vi "Set Transfer Groups.vi"(6 "Async Tx Transfer Groups":refnum<class "Transfer Group.lvclass">[](array[class]), 8 "Async Rx Transfer Groups":refnum<class "Transfer Group.lvclass">[](array[class]), 9 "Inline Tx Transfer Groups":refnum<class "Transfer Group.lvclass">[](array[class]), 10 "Inline Rx Transfer Groups":refnum<class "Transfer Group.lvclass">[](array[class]), 11 "Mock Plugin in":refnum<class "Mock Plugin.lvclass">) -> (3 "Mock Plugin out":refnum<class "Mock Plugin.lvclass">)   [LabVIEW 2017, in "Mock Plugin.lvclass"]
uses:
  Mock Plugin.lvclass
  C:/github/data-sharing-framework/Data Sharing Framework Core/Engine/Classes/Plugin/Plugin.lvclass
  Engine/Classes/Transfer Group/Transfer Group.lvclass
  Engine/Classes/Plugin/Plugin.lvclass/Plugin.ctl
  Engine/Classes/Plugin/Plugin.lvclass
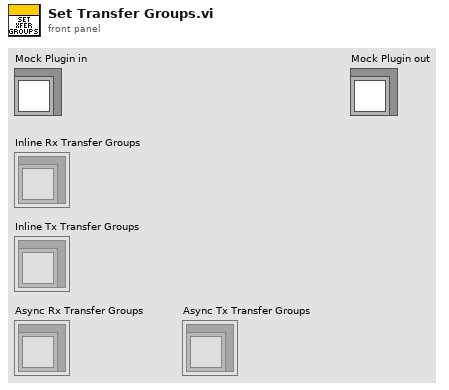
[diagram p1: front panel]
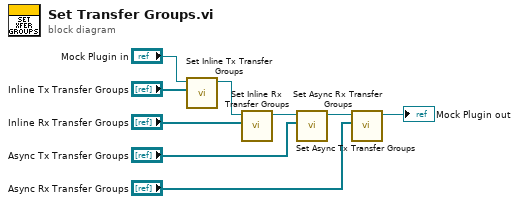
[diagram p0: block diagram]
diagram:
  n1 = call "Set Inline Tx Transfer Groups.vi"("Inline Tx Transfer Groups"="Inline Tx Transfer Groups", "Plugin in"="Mock Plugin in") -> ("Plugin out"=w7:refnum<class "Mock Plugin.lvclass">)  [unwired: 9 in]
  n2 = call "Set Inline Rx Transfer Groups.vi"("Inline Rx Transfer Groups"="Inline Rx Transfer Groups", "Plugin in"=w7) -> ("Plugin out"=w6:refnum<class "Mock Plugin.lvclass">)  [unwired: 9 in]
  n3 = call "Set Async Tx Transfer Groups.vi"("Async Tx Transfer Groups"="Async Tx Transfer Groups", "Plugin in"=w6) -> ("Plugin out"=w5:refnum<class "Mock Plugin.lvclass">)  [unwired: 9 in]
  n4 = call "Set Async Rx Transfer Groups.vi"("Async Rx Transfer Groups"="Async Rx Transfer Groups", "Plugin in"=w5) -> ("Plugin out"=→"Mock Plugin out":refnum<class "Mock Plugin.lvclass">)  [unwired: 9 in]
